vi "Delay.vi"(1 "error in (no error)":errorcluster, 4 "milliseconds to wait (1 ms)":u32=1, 8 "Enable? (T)":bool=TRUE) -> (15 "error out":errorcluster)   [LabVIEW 2011]
doc: "Insert a delay with error pass-through to provide data-flow control. Delays regardless of error in.\n\n\nVersion 1.0 - 10/21/2009\n\nPhaeron, Inc.\nwww.phaeron.com\ninfo@phaeron.com"
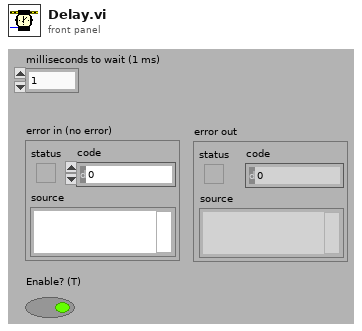
[diagram p1: front panel]
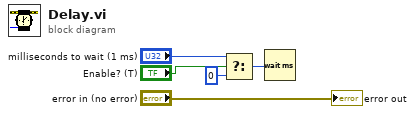
[diagram p0: block diagram]
diagram:
  n1 = Select(t="milliseconds to wait (1 ms)", s="Enable? (T)", f=u32 0) -> (s? t:f=w2:u32)
  n2 = Wait (ms)(milliseconds to wait=w2) -> ()  [unwired: 1 out]
  "error out" <- "error in (no error)"
